vi "interface in.vi"() -> (4 "time (global)":dbl, 8 "MPV":i32, 15 "global stop":bool)   [LabVIEW 2010, in "Licor-Steuerung.lvlib"]
uses:
  Licor-Steuerung.lvlib
  Licor-Sequences.ctl
  Johnny/pertrasgc fpga/gvbooleschRT.vi
  Johnny/pertrasgc fpga/GVVentilposition.vi
  Johnny/pertrasgc fpga/GVZeitenZyklen.vi
panel:
  out "Numerisch":i32
  out "sequence manual":T1=enum."WAIT"
  in  "sequence manual":T1=enum."warmup"
  out "sequence manual ?":bool
  in  "sequence manual ?":bool
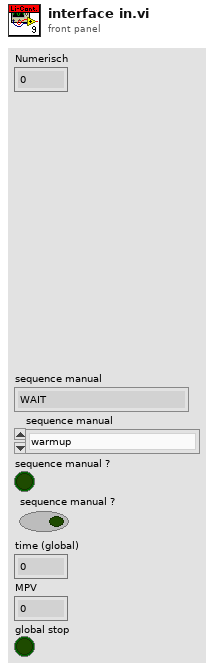
[diagram p1: front panel]
types:
  T1 = typedef "Licor-Steuerung.lvlib/Licor-Sequences.ctl" = enum16{"test", "WAIT", "warmup", "initialize", "calibrate Z", "calibrate S"}
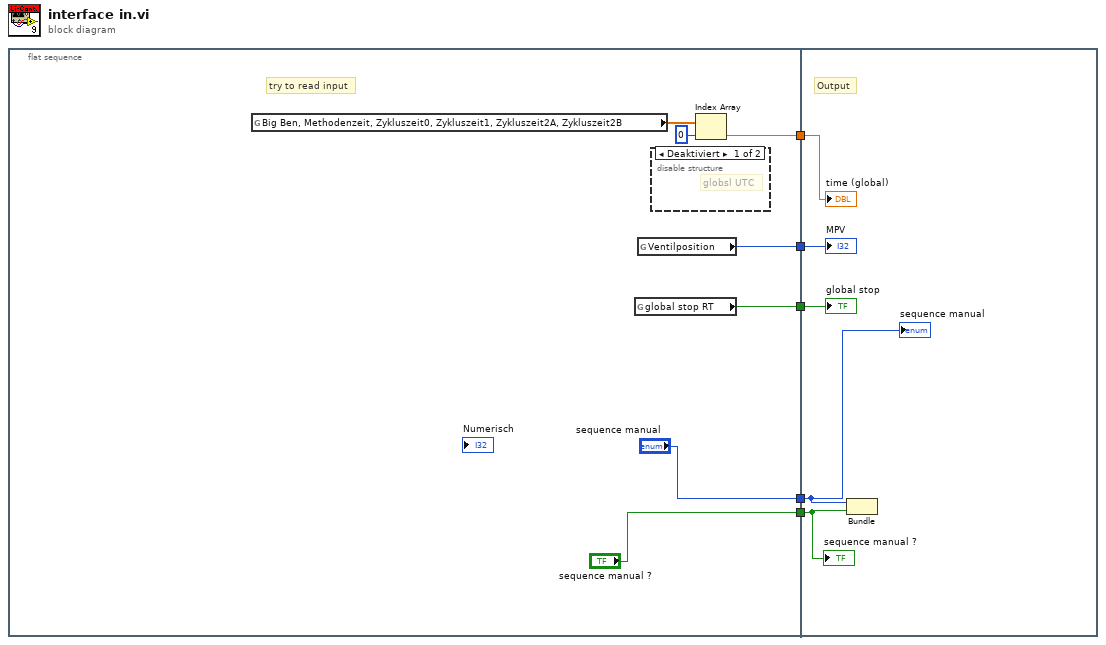
[diagram p0: block diagram]
diagram:
  n1 = flat-sequence {
    tunnel: [w12] -> w5
    tunnel: [w11] -> w4
    tunnel: ["sequence manual"] -> w3
    tunnel: ["sequence manual ?"] -> w2
    tunnel: [w6] -> w1
    tunnel: w5 -> [w17]
    tunnel: w4 -> [w16]
    tunnel: w3 -> [w15]
    tunnel: w2 -> [w14]
    tunnel: w1 -> [w13]
    frame #0 {
      # "try to read input"
      n2 = global read "GVZeitenZyklen.vi" "Big Ben, Methodenzeit, Zykluszeit0, Zykluszeit1, Zykluszeit2A, Zykluszeit2B"() -> (w9:dbl[])
      n3 = global read "gvbooleschRT.vi" "global stop RT"() -> (w11:bool)
      n4 = global read "GVVentilposition.vi" "Ventilposition"() -> (w12:i32)
      n5 = disable-structure shown="Deaktiviert" {
        frame Disabled {
          # "globsl UTC"
        }
        frame Enabled {
        }
      }
      n6 = Index Array(array=w9, index=0 ("Index")) -> (element=w6:dbl)
    }
    frame #1 {
      # "Output"
      n7 = Bundle("sequence manual"=w15, "sequence manual ?"=w14) -> ()  [unwired: 1 in, 1 out]
      "time (global)" <- w13
      "MPV" <- w17
      "global stop" <- w16
      "sequence manual ?" <- w14
      "sequence manual" <- w15
    }
  }
